vi "HTS_CHANGE_PMC_COMMANDS.vi"(7 "Loader Settings":T1={"Sample Flow Rate (uL/s)"=10.0, "Sample Volume (uL)"=80.0, "Mixing Volume (uL)"=200, "Mixing Speed (uL/s)"=1, "Mix#"=5, "Wash Volume (uL)"=100, "INJECTION_MODE"=enum."HT"} {"Sample Volume (uL)" min=2.0 max=200.0 step=0.5; "Mixing Volume (uL)" min=5 max=100 step=5; "Mixing Speed (uL/s)" min=25 max=250 step=5; "Sample Flow Rate (uL/s)" min=0.5 max=3.0 step=0.5 format="%_2f"; "Mix#" min=0 max=5 step=1; "Wash Volume (uL)" min=200 max=800 step=20}, 8 "Error IN":errorcluster, 10 "HTS_PMC_COMMAND_LIST":string[][](array[string])) -> (0 "Error OUT":errorcluster, 2 "NEW_PMC_COMMANDS":string[][](array[string]))   [LabVIEW 2009]
uses:
  HTS_LOADER_SETTINGS.ctl
  HTS_INJECTION_MODE.ctl
  HTS_PMC_COMMAND.ctl
  HTS_CAVRO_COMMAND.ctl
  HTS_CAVRO_COMMAND_TYPE.ctl
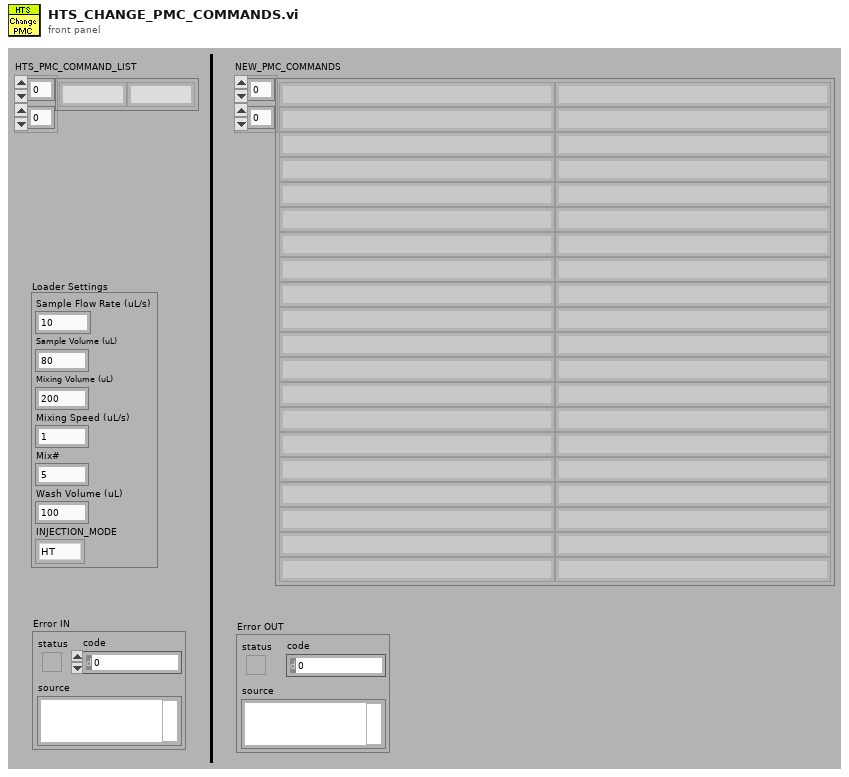
[diagram p1: front panel]
types:
  T1 = typedef "HTS_LOADER_SETTINGS.ctl" = cluster{"Sample Flow Rate (uL/s)":dbl, "Sample Volume (uL)":dbl, "Mixing Volume (uL)":i32, "Mixing Speed (uL/s)":i32, "Mix#":i32, "Wash Volume (uL)":i32, "INJECTION_MODE":T2}
  T2 = typedef "HTS_INJECTION_MODE.ctl" = enum16{"STD", "HT"}
  T3 = typedef "HTS_PMC_COMMAND.ctl" = enum16{"INITIALIZE Pump #1", "PRIME Pump #1", "Get Status", "STOP", "FLUSH", "REFILL Pump #1", "Last Flush and Refill", "MIX", "BOOST", "ACQUIRE and PURGE Pump #1", "ASPIRATE  an Air Bubble before lowering into the second or later well", "ASPIRATE from a well", "ASPIRATE an air bubble while moving", "ASPIRATE an air bubble before lowering probe into the injection port", "INITIALIZE Pump #2", "Move valve #2 of Pump #2", "PRIME Pump #2", "ACQUIRE Pump #2", "REFILL Pump #2", "PURGE Pump #2", "Cover Error Pump #1", "Cover Error Pump #2", "Pressure Error Pump #1", "Pressure Error Pump #2", "Motion Error Pump #1", "Motion Error Pump #2", "STD timer expired pump #1", "STD timer expired pump #2", "HTS timer expired pump #1", "HTS timer expired pump #2"}
  T4 = typedef "HTS_CAVRO_COMMAND.ctl" = cluster{"COMMAND":T5, "Parameter <n>":i32}
  T5 = typedef "HTS_CAVRO_COMMAND_TYPE.ctl" = enum16{"Move valve to INPUT", "Move valve to INPUT <n>", "Move valve to OUTPUT", "Move valve to OUTPUT <n>", "Move valve to BYPASS", "Move valve to EXTRA", "Syringe to ABSOLUTE  <n>", "Syringe RELATIVE Pickup <n>", "Syringe RELATIVE Dispense <n>", "Set START SPEED <n>", "Set TOP SPEED <n>", "Set CUTOFF in pulses/sec <n>", "Set CUTOFF in increments <n>", "Set SLOPE <n>", "Loop START", "Loop END <n>", "Set AUX OUTPUT <n>", "Delay Command Execution <n>", "EXECUTE COMMAND"}
  T6 = cluster{"Sample Flow Rate (uL/s)":dbl, "Sample Volume (uL)":dbl, "Mixing Volume (uL)":i32, "Mixing Speed (uL/s)":i32, "Mix#":i32, "Wash Volume (uL)":i32, "INJECTION_MODE":i32}
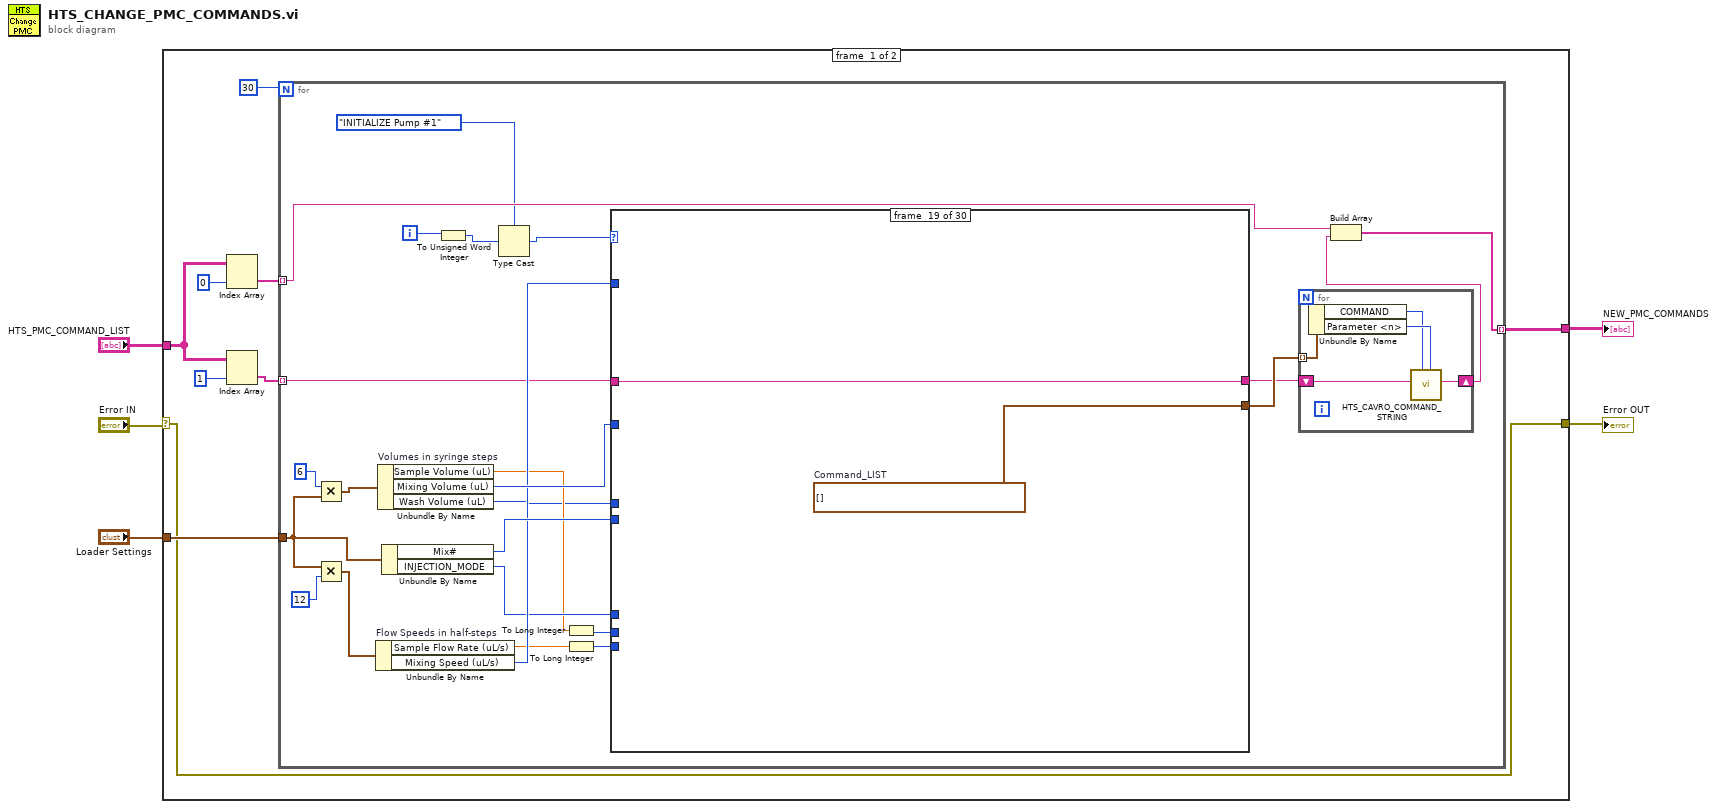
[diagram p0: block diagram]
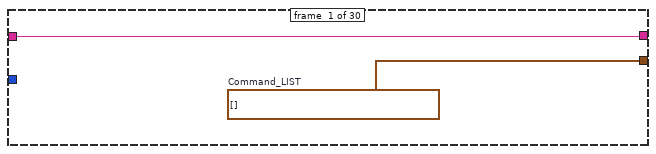
[diagram p2: hidden frame]
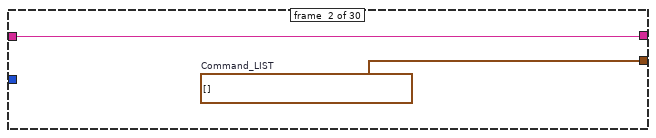
[diagram p3: hidden frame]
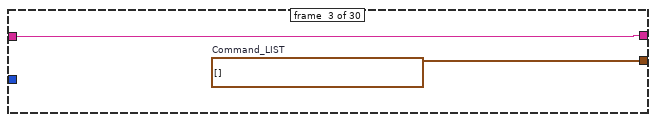
[diagram p4: hidden frame]
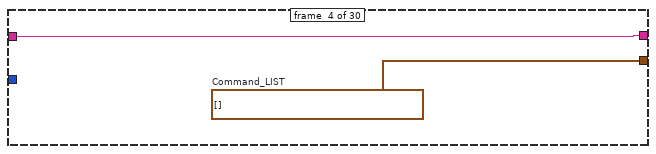
[diagram p5: hidden frame]
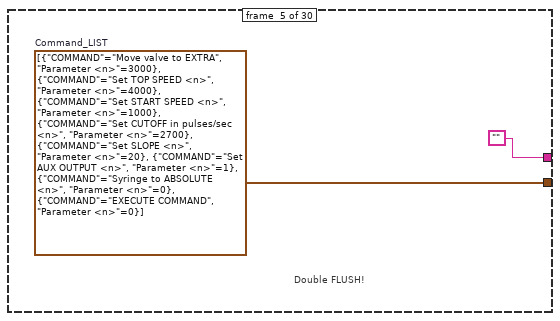
[diagram p6: hidden frame]
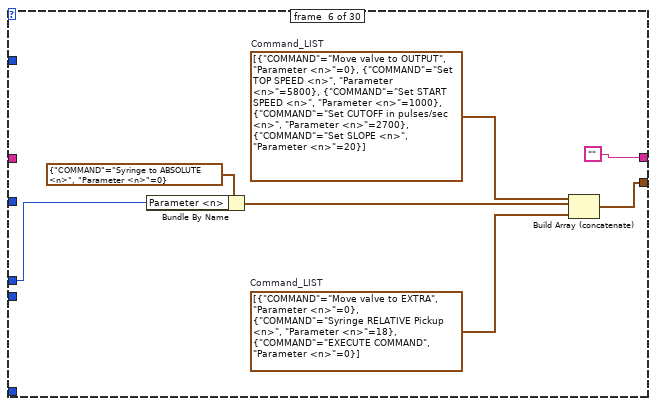
[diagram p7: hidden frame]
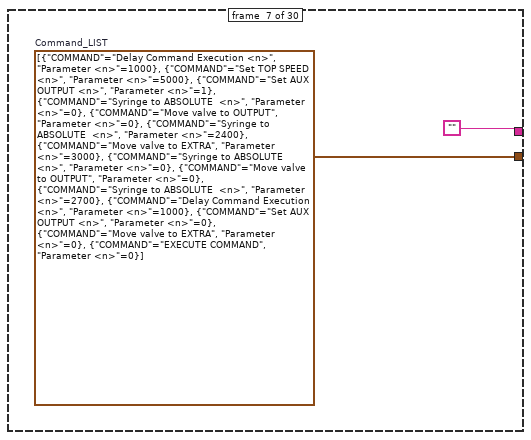
[diagram p8: hidden frame]
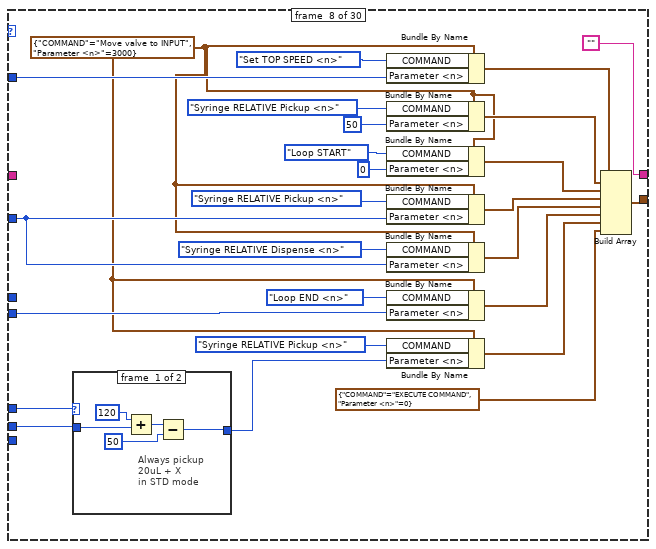
[diagram p9: hidden frame]
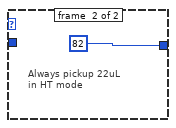
[diagram p10: hidden frame]
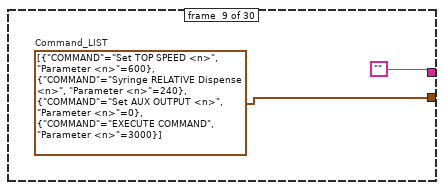
[diagram p11: hidden frame]
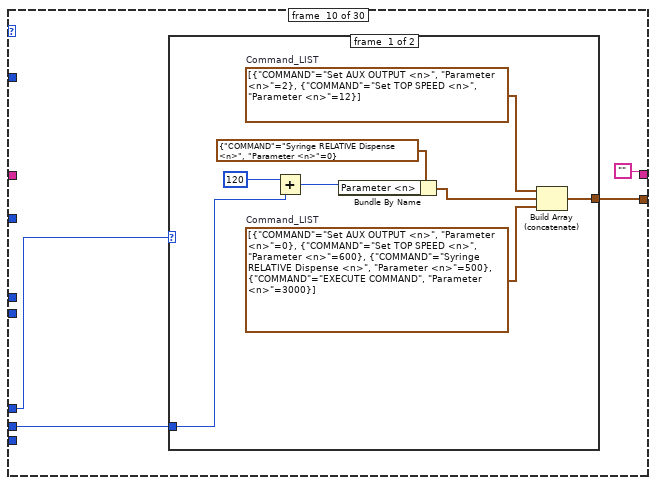
[diagram p12: hidden frame]
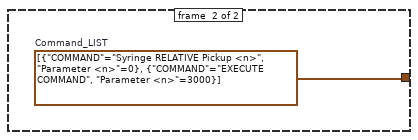
[diagram p13: hidden frame]
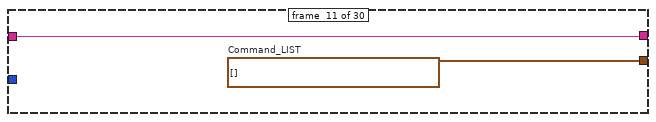
[diagram p14: hidden frame]
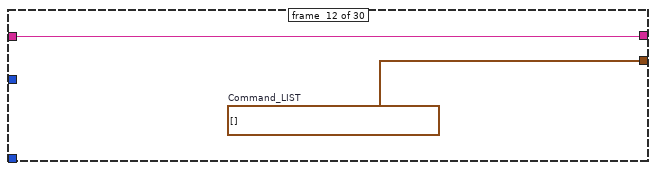
[diagram p15: hidden frame]
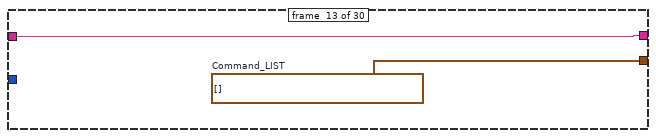
[diagram p16: hidden frame]
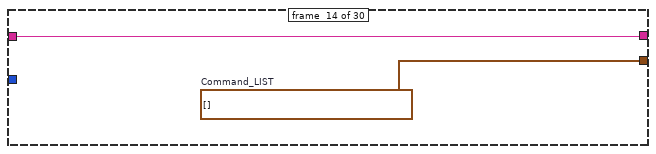
[diagram p17: hidden frame]
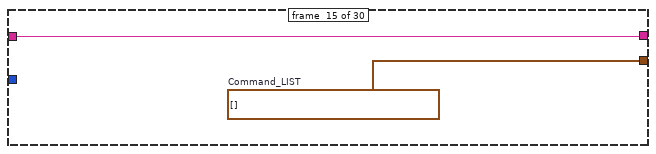
[diagram p18: hidden frame]
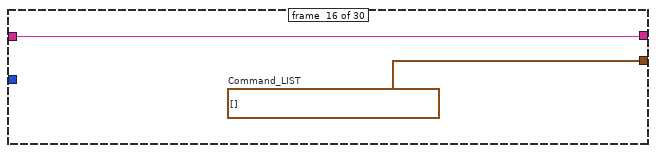
[diagram p19: hidden frame]
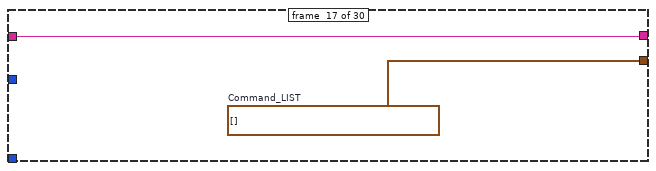
[diagram p20: hidden frame]
diagram:
  n1 = case shown="No Error" "Error IN" {
    selector: "Error IN" -> [w6 w163]
    tunnel: "Loader Settings" -> [w13 _]
    tunnel: [w8 w164] -> w4
    tunnel: "HTS_PMC_COMMAND_LIST" -> [w7 w164]
    tunnel: [w6 w163] -> w1
    frame #0 {
      n2 = Index Array(array=w7, index (col)=0 ("disabled index (col)")) -> (element=w9:string[])  [unwired: 1 in]
      n3 = Index Array(array=w7, index (col)=1 ("disabled index (col)")) -> (element=w12:string[])  [unwired: 1 in]
      n4 = for {
        N: 30 -> [_]
        tunnel: [w36] -> w8 mode=indexing
        tunnel: w13 -> [w30]
        tunnel: w12 -> [w18] mode=indexing
        tunnel: w9 -> [w16] mode=indexing
        i -> [w19]
        n5 = Multiply(x=6, y=w30) -> (x*y=w31:T6)
        n6 = Multiply(x=w30, y=12) -> (x*y=w34:T6)
        n7 = Unbundle By Name "Flow Speeds in half-steps"(w34) -> ("Sample Flow Rate (uL/s)"=w22:dbl, "Mixing Speed (uL/s)"=w27:i32)
        n8 = Unbundle By Name "Volumes in syringe steps"(w31) -> ("Sample Volume (uL)"=w25:dbl, "Mixing Volume (uL)"=w28:i32, "Wash Volume (uL)"=w23:i32)
        n9 = Unbundle By Name(w30) -> ("Mix#"=w29:i32, "INJECTION_MODE"=w26:T2)
        n10 = To Unsigned Word Integer(number=w19) -> (unsigned 16bit integer=w37:u16)
        n11 = Type Cast(type=HTS_PMC_COMMAND."INITIALIZE Pump #1" ("HTS_PMC_COMMAND"), x=w37) -> (*(type *) &x=w38:T3)
        n12 = To Long Integer(number=w25) -> (32bit integer=w24:i32)
        n13 = To Long Integer(number=w22) -> (32bit integer=w21:i32)
        n14 = case shown="\"FLUSH\"" w38 {
          tunnel: [w45 w47 w49 w51 w53 w60 w62 w80 w96 w100 w111 w113 w115 w117 w119 w121 w123 w128 w140 w142 w144 w146 w148 w150 w152 w154 w156 w158 w160 w162] -> w32
          tunnel: w29 -> [_ _ _ _ _ _ _ w85 _ _ _ _ _ _ _ _ _ _ _ _ _ _ _ _ _ _ _ _ _ _]
          tunnel: w28 -> [_ _ _ _ _ _ _ w84 _ _ _ _ _ _ _ _ _ _ _ _ _ _ _ _ _ _ _ _ _ _]
          tunnel: w27 -> [_ _ _ _ _ _ _ w76 _ _ _ _ _ _ _ _ _ _ _ _ _ _ _ _ _ _ _ _ _ _]
          tunnel: w26 -> [_ _ _ _ _ _ _ w70 _ w97 _ _ _ _ _ _ _ w127 _ _ _ _ _ _ _ _ _ _ _ _]
          tunnel: w24 -> [_ _ _ _ _ _ _ w66 _ w99 _ _ _ _ _ _ _ w125 _ _ _ _ _ _ _ _ _ _ _ _]
          tunnel: w23 -> [_ _ _ _ _ w56 _ _ _ _ _ _ _ _ _ _ _ _ _ _ _ _ _ _ _ _ _ _ _ _]
          tunnel: w21 -> [_ _ _ _ _ _ _ _ _ _ _ _ _ _ _ _ _ w126 _ _ _ _ _ _ _ _ _ _ _ _]
          tunnel: [w44 w46 w48 w50 "" "" "" "" "" "" w110 w112 w114 w116 w118 w120 w122 "" w139 w141 w143 w145 w147 w149 w151 w153 w155 w157 w159 w161] -> w17
          tunnel: w18 -> [w44 w46 w48 w50 _ _ _ _ _ _ w110 w112 w114 w116 w118 w120 w122 _ w139 w141 w143 w145 w147 w149 w151 w153 w155 w157 w159 w161]
          frame #0 {
            w45 = T4[] []  # Command_LIST
          }
          frame #1 {
            w47 = T4[] []  # Command_LIST
          }
          frame #2 {
            w49 = T4[] []  # Command_LIST
          }
          frame #3 {
            w51 = T4[] []  # Command_LIST
          }
          frame #4 {
            w53 = T4[] [{"COMMAND"=enum."Move valve to EXTRA", "Parameter <n>"=3000}, {"COMMAND"=enum."Set TOP SPEED <n>", "Parameter <n>"=4000}, {"COMMAND"=enum."Set START SPEED <n>", "Parameter <n>"=1000}, {"COMMAND"=enum."Set CUTOFF in pulses/sec <n>", "Parameter <n>"=2700}, {"COMMAND"=enum."Set SLOPE <n>", "Parameter <n>"=20}, {"COMMAND"=enum."Set AUX OUTPUT <n>", "Parameter <n>"=1}, {"COMMAND"=enum."Syringe to ABSOLUTE  <n>", "Parameter <n>"=0}, {"COMMAND"=enum."EXECUTE COMMAND", "Parameter <n>"=0}]  # Command_LIST
            # "Double FLUSH!"
          }
          frame #5 {
            w58 = T4[] [{"COMMAND"=enum."Move valve to EXTRA", "Parameter <n>"=0}, {"COMMAND"=enum."Syringe RELATIVE Pickup <n>", "Parameter <n>"=18}, {"COMMAND"=enum."EXECUTE COMMAND", "Parameter <n>"=0}]  # Command_LIST
            w59 = T4[] [{"COMMAND"=enum."Move valve to OUTPUT", "Parameter <n>"=0}, {"COMMAND"=enum."Set TOP SPEED <n>", "Parameter <n>"=5800}, {"COMMAND"=enum."Set START SPEED <n>", "Parameter <n>"=1000}, {"COMMAND"=enum."Set CUTOFF in pulses/sec <n>", "Parameter <n>"=2700}, {"COMMAND"=enum."Set SLOPE <n>", "Parameter <n>"=20}]  # Command_LIST
            n15 = Bundle By Name(cluster=T4 {"COMMAND"=enum."Syringe to ABSOLUTE  <n>", "Parameter <n>"=0} ("CAVRO_COMMAND"), "Parameter <n>"=w56) -> (w55:T4)
            n16 = Build Array (concatenate)(w59, w55, w58) -> (w60:T4[])
          }
          frame #6 {
            w62 = T4[] [{"COMMAND"=enum."Delay Command Execution <n>", "Parameter <n>"=1000}, {"COMMAND"=enum."Set TOP SPEED <n>", "Parameter <n>"=5000}, {"COMMAND"=enum."Set AUX OUTPUT <n>", "Parameter <n>"=1}, {"COMMAND"=enum."Syringe to ABSOLUTE  <n>", "Parameter <n>"=0}, {"COMMAND"=enum."Move valve to OUTPUT", "Parameter <n>"=0}, {"COMMAND"=enum."Syringe to ABSOLUTE  <n>", "Parameter <n>"=2400}, {"COMMAND"=enum."Move valve to EXTRA", "Parameter <n>"=3000}, {"COMMAND"=enum."Syringe to ABSOLUTE  <n>", "Parameter <n>"=0}, {"COMMAND"=enum."Move valve to OUTPUT", "Parameter <n>"=0}, {"COMMAND"=enum."Syringe to ABSOLUTE  <n>", "Parameter <n>"=2700}, {"COMMAND"=enum."Delay Command Execution <n>", "Parameter <n>"=1000}, {"COMMAND"=enum."Set AUX OUTPUT <n>", "Parameter <n>"=0}, {"COMMAND"=enum."Move valve to EXTRA", "Parameter <n>"=0}, {"COMMAND"=enum."EXECUTE COMMAND", "Parameter <n>"=0}]  # Command_LIST
          }
          frame #7 {
            w64 = T4 {"COMMAND"=enum."Move valve to INPUT", "Parameter <n>"=3000} ("CAVRO_COMMAND")
            n17 = case shown="\"STD\", Default" w70 {
              tunnel: [w92 82 ("Parameter <n>")] -> w67
              tunnel: w66 -> [w91 _]
              frame #0 {
                # "Always pickup\n20uL + X\nin STD mode"
                n18 = Add(x=120, y=w91) -> (x+y=w90:i32)
                n19 = Subtract(x=w90, y=50 ("Parameter <n>")) -> (x-y=w92:i32)
              }
              frame #1 {
                # "Always pickup 22uL\nin HT mode"
              }
            }
            n20 = Bundle By Name(cluster=w64, "COMMAND"=HTS_CAVRO_COMMAND_TYPE."Set TOP SPEED <n>", "Parameter <n>"=w76) -> (w71:T4)
            n21 = Bundle By Name(cluster=w64, "COMMAND"=HTS_CAVRO_COMMAND_TYPE."Syringe RELATIVE Pickup <n>", "Parameter <n>"=50) -> (w72:T4)
            n22 = Bundle By Name(cluster=w64, "COMMAND"=HTS_CAVRO_COMMAND_TYPE."Loop START", "Parameter <n>"=0) -> (w73:T4)
            n23 = Bundle By Name(cluster=w64, "COMMAND"=HTS_CAVRO_COMMAND_TYPE."Syringe RELATIVE Pickup <n>", "Parameter <n>"=w84) -> (w83:T4)
            n24 = Bundle By Name(cluster=w64, "COMMAND"=HTS_CAVRO_COMMAND_TYPE."Syringe RELATIVE Dispense <n>", "Parameter <n>"=w84) -> (w82:T4)
            n25 = Bundle By Name(cluster=w64, "COMMAND"=HTS_CAVRO_COMMAND_TYPE."Loop END <n>", "Parameter <n>"=w85) -> (w81:T4)
            n26 = Bundle By Name(cluster=w64, "COMMAND"=HTS_CAVRO_COMMAND_TYPE."Syringe RELATIVE Pickup <n>", "Parameter <n>"=w67) -> (w69:T4)
            n27 = Build Array(w71, w72, w73, w83, w82, w81, w69, T4 {"COMMAND"=enum."EXECUTE COMMAND", "Parameter <n>"=0} ("CAVRO_COMMAND")) -> (w80:T4[])
          }
          frame #8 {
            w96 = T4[] [{"COMMAND"=enum."Set TOP SPEED <n>", "Parameter <n>"=600}, {"COMMAND"=enum."Syringe RELATIVE Dispense <n>", "Parameter <n>"=240}, {"COMMAND"=enum."Set AUX OUTPUT <n>", "Parameter <n>"=0}, {"COMMAND"=enum."EXECUTE COMMAND", "Parameter <n>"=3000}]  # Command_LIST
          }
          frame #9 {
            n28 = case shown="\"STD\", Default" w97 {
              tunnel: [w107 w109] -> w100
              tunnel: w99 -> [w102 _]
              frame #0 {
                w104 = T4[] [{"COMMAND"=enum."Set AUX OUTPUT <n>", "Parameter <n>"=0}, {"COMMAND"=enum."Set TOP SPEED <n>", "Parameter <n>"=600}, {"COMMAND"=enum."Syringe RELATIVE Dispense <n>", "Parameter <n>"=500}, {"COMMAND"=enum."EXECUTE COMMAND", "Parameter <n>"=3000}]  # Command_LIST
                w106 = T4[] [{"COMMAND"=enum."Set AUX OUTPUT <n>", "Parameter <n>"=2}, {"COMMAND"=enum."Set TOP SPEED <n>", "Parameter <n>"=12}]  # Command_LIST
                n29 = Add(x=120, y=w102) -> (x+y=w103:i32)
                n30 = Bundle By Name(cluster=T4 {"COMMAND"=enum."Syringe RELATIVE Dispense <n>", "Parameter <n>"=0} ("CAVRO_COMMAND"), "Parameter <n>"=w103) -> (w105:T4)
                n31 = Build Array (concatenate)(w106, w105, w104) -> (w107:T4[])
              }
              frame #1 {
                w109 = T4[] [{"COMMAND"=enum."Syringe RELATIVE Pickup <n>", "Parameter <n>"=0}, {"COMMAND"=enum."EXECUTE COMMAND", "Parameter <n>"=3000}]  # Command_LIST
              }
            }
          }
          frame #10 {
            w111 = T4[] []  # Command_LIST
          }
          frame #11 {
            w113 = T4[] []  # Command_LIST
          }
          frame #12 {
            w115 = T4[] []  # Command_LIST
          }
          frame #13 {
            w117 = T4[] []  # Command_LIST
          }
          frame #14 {
            w119 = T4[] []  # Command_LIST
          }
          frame #15 {
            w121 = T4[] []  # Command_LIST
          }
          frame #16 {
            w123 = T4[] []  # Command_LIST
          }
          frame #17 {
            n32 = case shown="\"HT\"" w127 {
              tunnel: [w129 w137] -> w128
              tunnel: w126 -> [_ w133]
              tunnel: w125 -> [_ w131]
              frame #0 {
                w129 = T4[] [{"COMMAND"=enum."Syringe RELATIVE Pickup <n>", "Parameter <n>"=0}, {"COMMAND"=enum."EXECUTE COMMAND", "Parameter <n>"=0}]  # Command_LIST
              }
              frame #1 {
                w136 = T4[] [{"COMMAND"=enum."Set AUX OUTPUT <n>", "Parameter <n>"=0}, {"COMMAND"=enum."Set TOP SPEED <n>", "Parameter <n>"=600}, {"COMMAND"=enum."Syringe RELATIVE Dispense <n>", "Parameter <n>"=120}, {"COMMAND"=enum."EXECUTE COMMAND", "Parameter <n>"=3000}]  # Command_LIST
                w138 = T4[] [{"COMMAND"=enum."Move valve to OUTPUT", "Parameter <n>"=0}, {"COMMAND"=enum."Set AUX OUTPUT <n>", "Parameter <n>"=1}, {"COMMAND"=enum."Set TOP SPEED <n>", "Parameter <n>"=120}, {"COMMAND"=enum."Syringe RELATIVE Dispense <n>", "Parameter <n>"=12}]  # Command_LIST
                n33 = Bundle By Name(cluster=T4 {"COMMAND"=enum."Set TOP SPEED <n>", "Parameter <n>"=0} ("CAVRO_COMMAND"), "Parameter <n>"=w133) -> (w134:T4)
                n34 = Bundle By Name(cluster=T4 {"COMMAND"=enum."Syringe RELATIVE Dispense <n>", "Parameter <n>"=0} ("CAVRO_COMMAND"), "Parameter <n>"=w131) -> (w130:T4)
                n35 = Build Array (concatenate)(w138, w134, w130, w136) -> (w137:T4[])
              }
            }
          }
          frame #18 {
            w140 = T4[] []  # Command_LIST
          }
          frame #19 {
            w142 = T4[] []  # Command_LIST
          }
          frame #20 {
            w144 = T4[] []  # Command_LIST
          }
          frame #21 {
            w146 = T4[] []  # Command_LIST
          }
          frame #22 {
            w148 = T4[] []  # Command_LIST
          }
          frame #23 {
            w150 = T4[] []  # Command_LIST
          }
          frame #24 {
            w152 = T4[] []  # Command_LIST
          }
          frame #25 {
            w154 = T4[] []  # Command_LIST
          }
          frame #26 {
            w156 = T4[] []  # Command_LIST
          }
          frame #27 {
            w158 = T4[] []  # Command_LIST
          }
          frame #28 {
            w160 = T4[] []  # Command_LIST
          }
          frame #29 {
            w162 = T4[] []  # Command_LIST
          }
        }
        n36 = for {
          shift-right: [w42] -> w20
          shift-left: w17 -> [w43]
          tunnel: w32 -> [w39] mode=indexing
          n37 = Unbundle By Name(w39) -> ("COMMAND"=w40:T5, "Parameter <n>"=w41:i32)
          n38 = call "HTS_CAVRO_COMMAND_STRING.vi"("Prior Command"=w43, "PUMP COMMAND"=w40, "Parameter <n>"=w41) -> ("New Command"=w42:string)  [unwired: 4 out]
        }
        n39 = Build Array(w16, w20) -> (w36:string[])
      }
    }
    frame #1 {
    }
  }
  "NEW_PMC_COMMANDS" <- w4
  "Error OUT" <- w1
